vi "Save_Waveforms.vi"(7 "Cluster":T1 {"File Location" items=["Unknown"=-1, "Storage"=0, "Processing"=1, "Unmerged"=2]; "Estimate Source" items=["Any Source."=-2, "No Shot"=-1, "Basic Labview Estimate"=0, "IDL Estimate From Andrew"=1, "IDL Estimate From Tobin"=2, "Old Metadata"=3]}, 8 "error in (no error)":errorcluster, 10 "id_dust_event":i64, 11 "ref":i32) -> (0 "error out":errorcluster, 3 "ref out":i32)   [LabVIEW 2013]
uses:
  <userlib>/Accelerator/User Interface/Controls/Query_Dust_Event.ctl
  <userlib>/Accelerator/User Interface/Controls/Estimate_source.ctl
  <userlib>/Accelerator/User Interface/Controls/File_location.ctl
  <vilib>/addons/h5labview/H5F_mode.ctl
  <userlib>/_OpenG.lib/file/file.llb/File Exists - Scalar__ogtk.vi
  <vilib>/addons/h5labview/H5File.lvlib
  <vilib>/addons/h5labview/H5GroupObject.lvlib
panel:
  # "Dust Event"
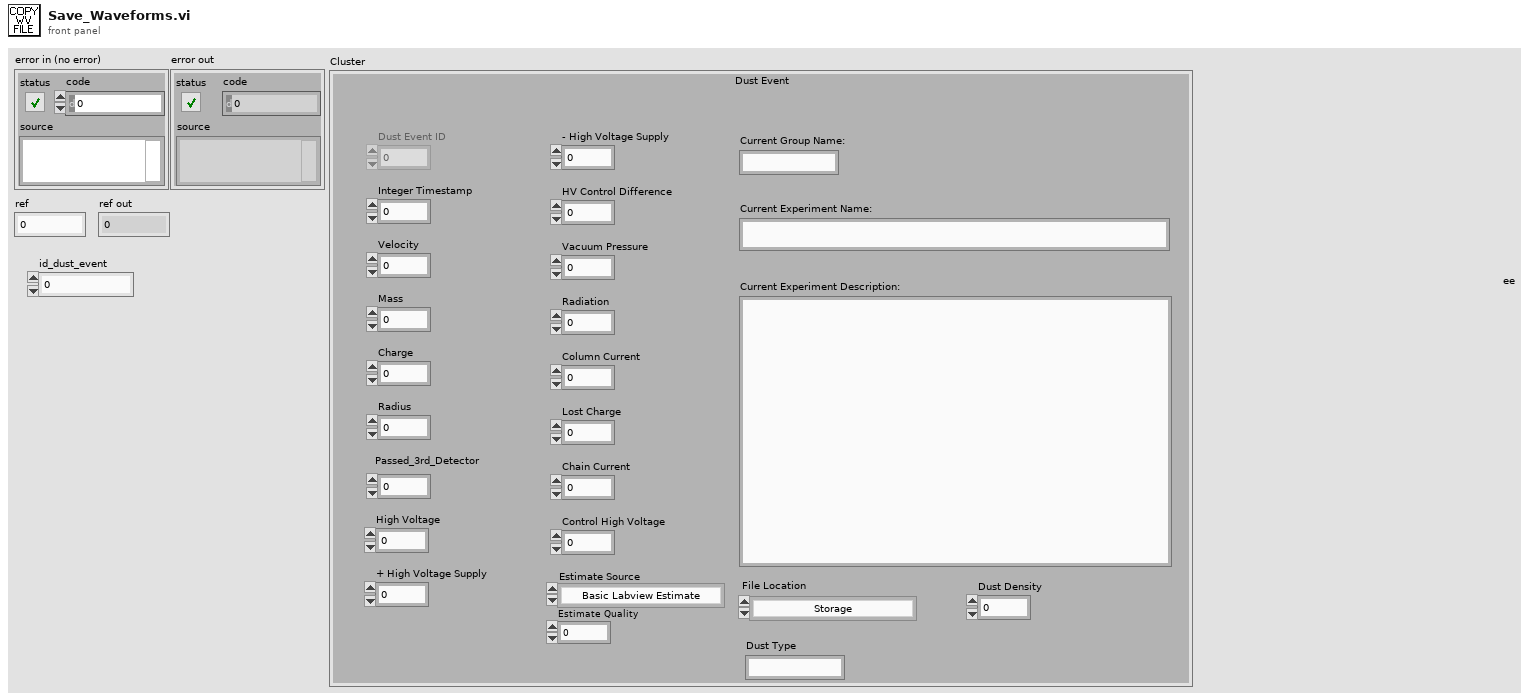
[diagram p1: front panel]
types:
  T1 = typedef "Query_Dust_Event.ctl" = cluster{"Dust Event ID":i64, "Integer Timestamp":i64, "Velocity":dbl, "Mass":dbl, "Charge":sgl, "Radius":sgl, "Passed_3rd_Detector":i8, "High Voltage":sgl, "+ High Voltage Supply":sgl, "- High Voltage Supply":sgl, "HV Control Difference":sgl, "Vacuum Pressure":sgl, "Radiation":sgl, "Column Current":sgl, "Lost Charge":sgl, "Chain Current":sgl, "Control High Voltage":sgl, "Current Group Name:":string, "Current Experiment Name:":string, "Current Experiment Description:":string, "Estimate Source":T2, "Estimate Quality":i8, "File Location":T3, "Dust Type":string, "Dust Density":sgl}
  T2 = typedef "Estimate_source.ctl" = i8
  T3 = typedef "File_location.ctl" = i8
  T4 = typedef "H5File.lvlib/H5F_mode.ctl" = enum16{"read-only", "read-write", "overwrite", "create new", "open or create"}
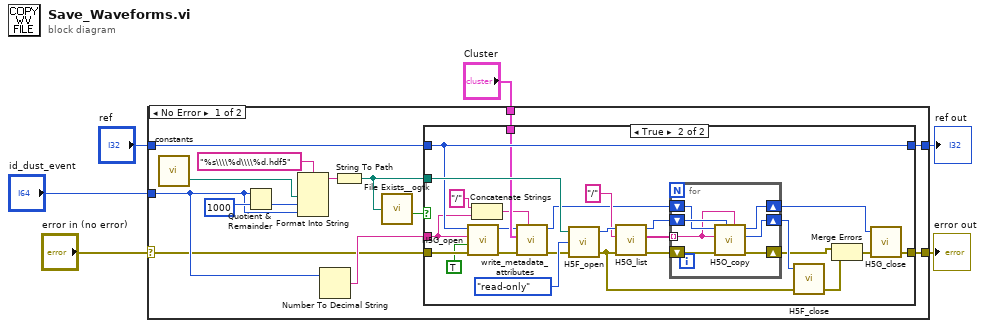
[diagram p0: block diagram]
diagram:
  n1 = case shown="No Error" "error in (no error)" {
    selector: "error in (no error)" -> [w7 w56]
    tunnel: [w13 w56] -> w4
    tunnel: "id_dust_event" -> [w12 _]
    tunnel: "ref" -> [w10 w55]
    tunnel: [w9 w55] -> w2
    tunnel: "Cluster" -> [w8 _]
    frame No Error {
      n2 = call <userlib>:"constants.vi"() -> ("Processed HDF5 filepath"=w18:path)  [unwired: 3 out]
      n3 = Quotient & Remainder(x=w12, y=i64 1000) -> (floor(x/y)=w17:i64)  [unwired: 1 out]
      n4 = Format Into String(format string="%s\\\\%d\\\\%d.hdf5", w18, w17, w12) -> (resulting string=w16:string)  [unwired: 2 in, 1 out]
      n5 = Number To Decimal String(number=w12) -> (decimal integer string=w11:string)  [unwired: 1 in]
      n6 = String To Path(string=w16) -> (path=w15:path)
      n7 = call-poly <userlib>:"File Exists__ogtk.vi"("file path"=w15) -> ("exists"=w14:bool)  [unwired: 6 in, 1 out]
      n8 = case shown="True" w14 {
        tunnel: w7 -> [w22 w39]
        tunnel: w15 -> [_ w46]
        tunnel: [w22 w37] -> w13
        tunnel: w10 -> [w21 w31]
        tunnel: [w21 w31] -> w9
        tunnel: w11 -> [_ w26]
        tunnel: w8 -> [_ w28]
        frame False {
        }
        frame True {
          n9 = call <vilib>:"H5G_open.vi"("error in (no error)"=w39, "create? (F)"=TRUE, "name"=w26, "ref"=w31) -> ("error out"=w30:errorcluster, "group"=w27:i32)  [unwired: 2 in]
          n10 = Concatenate Strings("/" ("string"), w26) -> (w24:string)
          n11 = call <userlib>:"write_metadata_attributes.vi"("Group ID"=w24, "error in (no error)"=w30, "Cluster"=w28, "group ref"=w27) -> ("error out"=w29:errorcluster, "group ref out"=w25:i32)  [unwired: 4 in]
          n12 = call <vilib>:"H5F_open.vi"("error in (no error)"=w29, "mode"=H5F_mode."read-only", "path"=w46) -> ("error out"=w35:errorcluster, "ref"=w45:i32)  [unwired: 1 in]
          n13 = call <vilib>:"H5G_list.vi"("error in (no error)"=w35, "group"="/", "ref"=w45) -> ("error out"=w44:errorcluster, "names"=w42:string[], "ref out"=w43:i32)  [unwired: 1 in, 1 out]
          n14 = for {
            shift-right: [w51] -> w32
            shift-left: w44 -> [w54]
            shift-right: [w52] -> w41
            shift-left: w43 -> [w53]
            tunnel: w42 -> [w48] mode=indexing
            shift-right: [w49] -> w36
            shift-left: w25 -> [w50]
            n15 = call <vilib>:"H5O_copy.vi"("src_name"=w48, "src_id"=w53, "error in (no error)"=w54, "dest_name"=w48, "dest_id"=w50) -> ("error out"=w51:errorcluster, "src out"=w52:i32, "dest out"=w49:i32)  [unwired: 4 in]
          }
          n16 = call <vilib>:"H5F_close.vi"("error in (no error)"=w35, "ref"=w41) -> ("error out"=w33:errorcluster)  [unwired: 3 in]
          n17 = Merge Errors(w32, w33) -> (w34:errorcluster)
          n18 = call <vilib>:"H5G_close.vi"("error in (no error)"=w34, "ref"=w36) -> ("error out"=w37:errorcluster)  [unwired: 3 in]
        }
      }
    }
    frame Error {
    }
  }
  "error out" <- w4
  "ref out" <- w2
